vi "Generate Digital Pulse.vi"(8 "error in (no error)":errorcluster, 9 "Approximate Pulse Width (s)":dbl=0.1 format="%#_13g", 10 "Channel":string="Aliases/Counter Writer", 11 "WorkspaceManager":T1) -> (0 "error out":errorcluster, 3 "Workspace Manager out":T1)   [LabVIEW 2016, in "Scan Engine cRIO System Tests.lvclass"]
uses:
  Scan Engine cRIO System Tests.lvclass
  <vilib>/NI Veristand/Execution/Workspace/WorkspaceAPI.ctl
  NationalInstruments.VeriStand.ClientAPI
  <vilib>/NI Veristand/Execution/Workspace/NI VeriStand - Set Single Channel Value.vi
  <vilib>/NI VeriStand/Execution/Workspace/NI_VS Workspace ExecutionAPI.lvlib
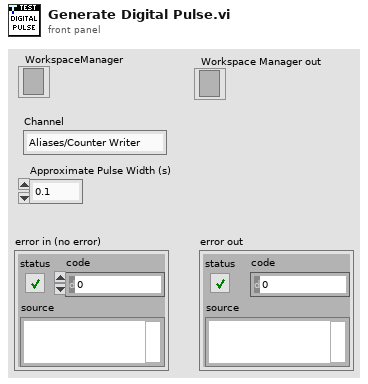
[diagram p1: front panel]
types:
  T1 = typedef "NI_VS Workspace ExecutionAPI.lvlib/WorkspaceAPI.ctl" = refnum<k24>
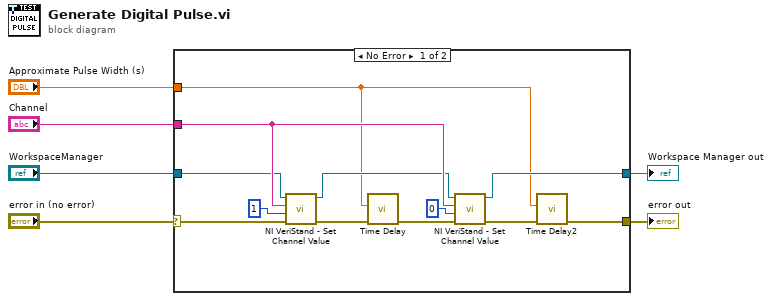
[diagram p0: block diagram]
diagram:
  n1 = case shown="No Error" "error in (no error)" {
    selector: "error in (no error)" -> [w12 w20]
    tunnel: "Channel" -> [w18 _]
    tunnel: [w17 w19] -> w5
    tunnel: [w16 w20] -> w4
    tunnel: "WorkspaceManager" -> [w8 w19]
    tunnel: "Approximate Pulse Width (s)" -> [w7 _]
    frame No Error {
      n2 = call-poly <vilib>:"NI VeriStand - Set Channel Value.vi"("error in (no error)"=w12, "Value"=1, "Channel"=w18, "WorkspaceManager in"=w8) -> ("error out"=w10:errorcluster, "WorkspaceManager out"=w9:T1)  [unwired: 6 in]
      n3 = call "Time Delay"("error in (no error)"=w10, "Delay Time (s)"=w7) -> ("error out"=w11:errorcluster)  [unwired: 9 in]
      n4 = call-poly <vilib>:"NI VeriStand - Set Channel Value.vi"("error in (no error)"=w11, "Value"=0, "Channel"=w18, "WorkspaceManager in"=w9) -> ("error out"=w15:errorcluster, "WorkspaceManager out"=w17:T1)  [unwired: 6 in]
      n5 = call "Time Delay2"("error in (no error)"=w15, "Delay Time (s)"=w7) -> ("error out"=w16:errorcluster)  [unwired: 9 in]
    }
    frame Error {
    }
  }
  "Workspace Manager out" <- w5
  "error out" <- w4
